vi "constructor.vi"(10 "Beverage.lvclass":refnum<class "Beverage.lvclass">, 11 "Mocha in":refnum<class "Mocha.lvclass">) -> (3 "Mocha out":refnum<class "Mocha.lvclass">)   [LabVIEW 2020, in "Mocha.lvclass"]
uses:
  Mocha.lvclass
  Beverage.lvclass
  Mocha.lvclass/Mocha.ctl
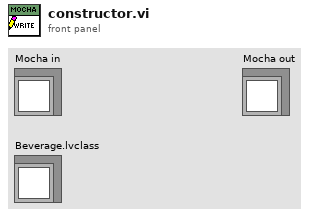
[diagram p1: front panel]
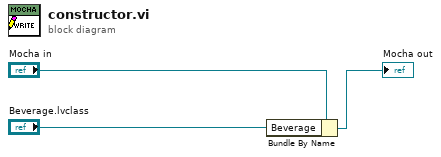
[diagram p0: block diagram]
diagram:
  n1 = Bundle By Name(cluster="Mocha in", "Beverage"="Beverage.lvclass") -> (→"Mocha out":refnum<class "Mocha.lvclass">)
